vi "8.10.1.vi"() -> ()   [LabVIEW 2018]
panel:
  out "수신 데이터":cluster{"이름":string, "토익 점수":dbl}
  in  "송신 데이터":cluster{"이름":string, "토익 점수":dbl}
  out "소비 루프 반복":dbl
  out "생산 루프 반복":dbl
  in  "정지":bool
  in  "데이터송신":bool
  # "Y"
  # "N"
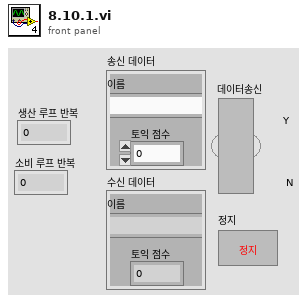
[diagram p1: front panel]
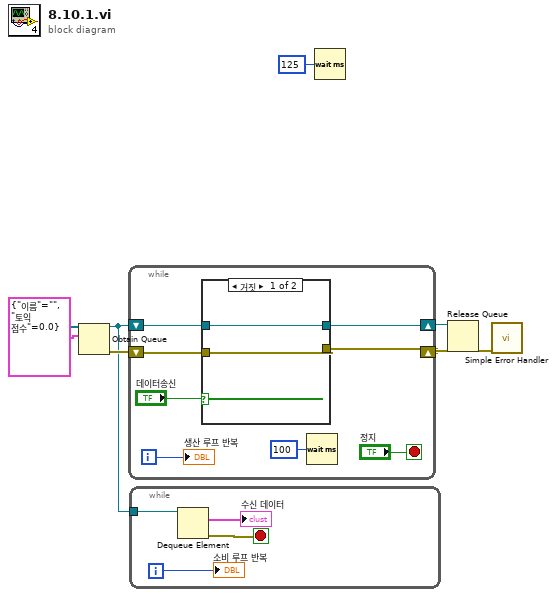
[diagram p0: block diagram]
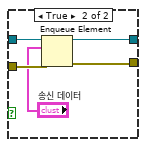
[diagram p2: hidden frame]
diagram:
  n1 = Obtain Queue(element data type=cluster{"이름":string, "토익 점수":dbl} {"이름"="", "토익 점수"=0.0} ("송신 데이터 2")) -> (queue out=w2:refnum<queue>, error out=w4:errorcluster)  [unwired: 4 in, 1 out]
  n2 = while {
    shift-right: [w10] -> w5
    shift-left: w2 -> [w11]
    shift-right: [w8] -> w3
    shift-left: w4 -> [w9]
    i -> [w15]
    stop <- "정지" stop-if-true
    n3 = case shown="거짓" "데이터송신" {
      tunnel: [w17 w21] -> w10
      tunnel: w11 -> [w17 w22]
      tunnel: [w16 w19] -> w8
      tunnel: w9 -> [w16 w20]
      frame False {
      }
      frame True {
        n4 = Enqueue Element(queue=w22, element="송신 데이터", error in (no error)=w20) -> (queue out=w21:refnum<queue>, error out=w19:errorcluster)  [unwired: 1 in, 1 out]
      }
    }
    n5 = Wait (ms)(milliseconds to wait=u32 100 ("대기 시간 (ms)")) -> ()  [unwired: 1 out]
    "생산 루프 반복" <- w15
  }
  n6 = while {
    tunnel: w2 -> [w25]
    i -> [w26]
    stop <- w23 stop-if-true
    n7 = Dequeue Element(queue=w25) -> (element=→"수신 데이터":cluster{"이름":string, "토익 점수":dbl}, error out=w23:errorcluster)  [unwired: 2 in, 2 out]
    "소비 루프 반복" <- w26
  }
  n8 = Wait (ms)(milliseconds to wait=u32 125 ("대기 시간 (ms)")) -> ()  [unwired: 1 out]
  n9 = Release Queue(queue=w5, error in (no error)=w3) -> (error out=w6:errorcluster)  [unwired: 1 in, 2 out]
  n10 = call <vilib>:"Simple Error Handler.vi"("error in (no error)"=w6) -> ()  [unwired: 4 in, 5 out]
